vi "OpenNodes.vi"(1 "Node Name":string) -> ()   [LabVIEW 2012]
doc: "If you do not wire in a node, it will open all running nodes - otherwise it will opent he node you requested."
uses:
  <userlib>/ROS for LabVIEW Software/ROS/Code/SubVIs/_ROSControl.ctl
  <userlib>/ROS for LabVIEW Software/ROS/Code/SubVIs/_ROSDirection.ctl
  <userlib>/ROS for LabVIEW Software/ROS/Code/_ROSDefinition.vi
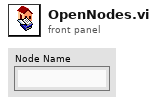
[diagram p1: front panel]
types:
  T1 = typedef "_ROSControl.ctl" = cluster{"topic port":u16, "Node":string, "topic":string, "type":string, "node port":u16, "error ":errorcluster, "Direction":T2, "Update (ms)":u16, "FIFO size":u16}
  T2 = typedef "_ROSDirection.ctl" = enum16{"Node", "Publisher", "Subscriber", "ServiceClient", "ServiceProvider"}
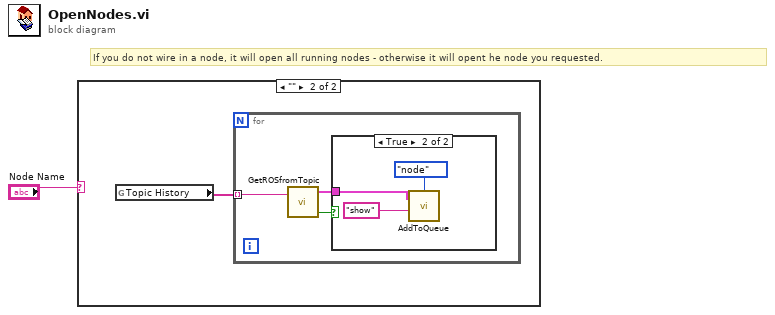
[diagram p0: block diagram]
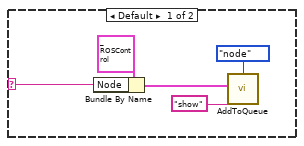
[diagram p2: hidden frame]
diagram:
  # "If you do not wire in a node, it will open all running nodes - otherwise it will opent he node you requested."
  n1 = case shown="\"\"" "Node Name" {
    selector: "Node Name" -> [w3 _]
    frame Default {
      n2 = Bundle By Name(cluster=T1 {"topic port"=0, "Node"="/fred", "topic"="/robot/head/command_head_nod", "type"="std_msgs/Bool", "node port"=59377, "error "={"status"=FALSE, "code"=0, "source"=""}, "Direction"=enum."Publisher", "Update (ms)"=1, "FIFO size"=1} ("ROS"), "Node"=w3) -> (w5:T1)
      n3 = call <userlib>:"AddToQueue.vi"("Cmd"="show" ("element"), "ROS"=w5, "Type"=enum16{"topic", "node", "ToFIFO", "ToWrite"}."node") -> ()  [unwired: 2 in, 1 out]
    }
    frame "" {
      n4 = global read "_ROSDefinition.vi" "Topic History"() -> (w7:string[])
      n5 = for {
        tunnel: w7 -> [w10] mode=indexing
        n6 = call <userlib>:"GetROSfromTopic.vi"("Topic"=w10) -> ("ROS"=w9:T1, "Node?"=w8:bool)  [unwired: 1 in, 1 out]
        n7 = case shown="True" w8 {
          tunnel: w9 -> [_ w12]
          frame False {
          }
          frame True {
            n8 = call <userlib>:"AddToQueue.vi"("Cmd"="show" ("element"), "ROS"=w12, "Type"=enum16{"topic", "node", "ToFIFO", "ToWrite"}."node") -> ()  [unwired: 2 in, 1 out]
          }
        }
      }
    }
  }
